vi "Create New IO Node.vi"(6 "Device Icon Name":string[](array[string]), 7 "Path to Analog Node Template":string="IONode\\Analog Input Node x.vi", 8 "error in":errorcluster, 9 "Device Alias":string, 10 "Values for Naming":T1={"Bus Number"=1, "Device Number"=1, "Channel Number"=1} {"Channel Number" min=1 step=1; "Device Number" min=1 step=1; "Bus Number" min=1 step=1}, 11 "Path to IO Node":path=path "D:/Documents/Projects/SPIAPI/IOEngineCode") -> (0 "error out":errorcluster, 2 "IO Node Name":string, 3 "Path to new IO Node":path)   [LabVIEW 2014, in "Initialization and IO Node Scripting.lvlib"]
uses:
  Initialization and IO Node Scripting.lvlib
  State Machine/Controls/Values for Naming.ctl
  Icon Editor/Icon Editor.llb/Icon Colors.ctl
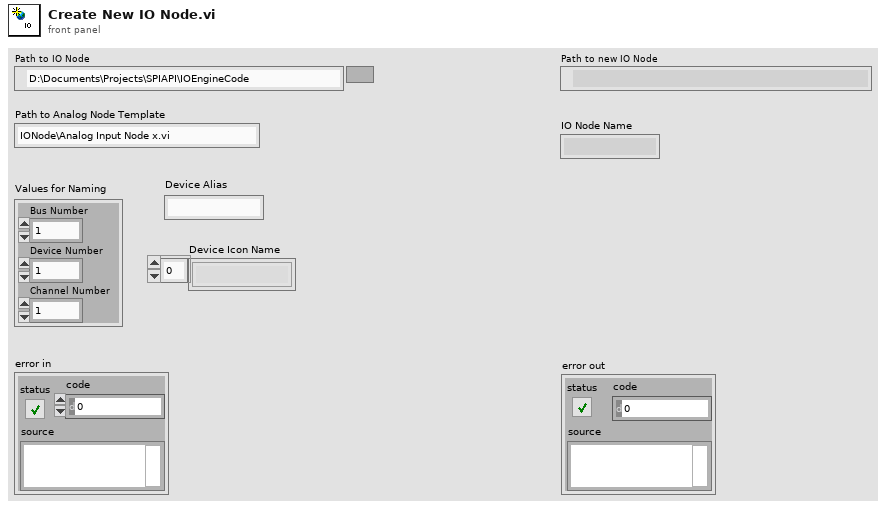
[diagram p1: front panel]
types:
  T1 = typedef "Initialization and IO Node Scripting.lvlib/Values for Naming.ctl" = cluster{"Bus Number":i32, "Device Number":i32, "Channel Number":i32}
  T2 = enum32{"invalid VI type", "Standard VI", "Control VI", "Global VI", "Polymorphic VI", "Configuration VI", "SubSystem", "Facade VI", "Method VI", "Statechart Diagram VI"}
  T3 = typedef "Initialization and IO Node Scripting.lvlib/Icon Colors.ctl" = cluster{"Text Color":u32, "Background Color":u32, "Border Color":u32}
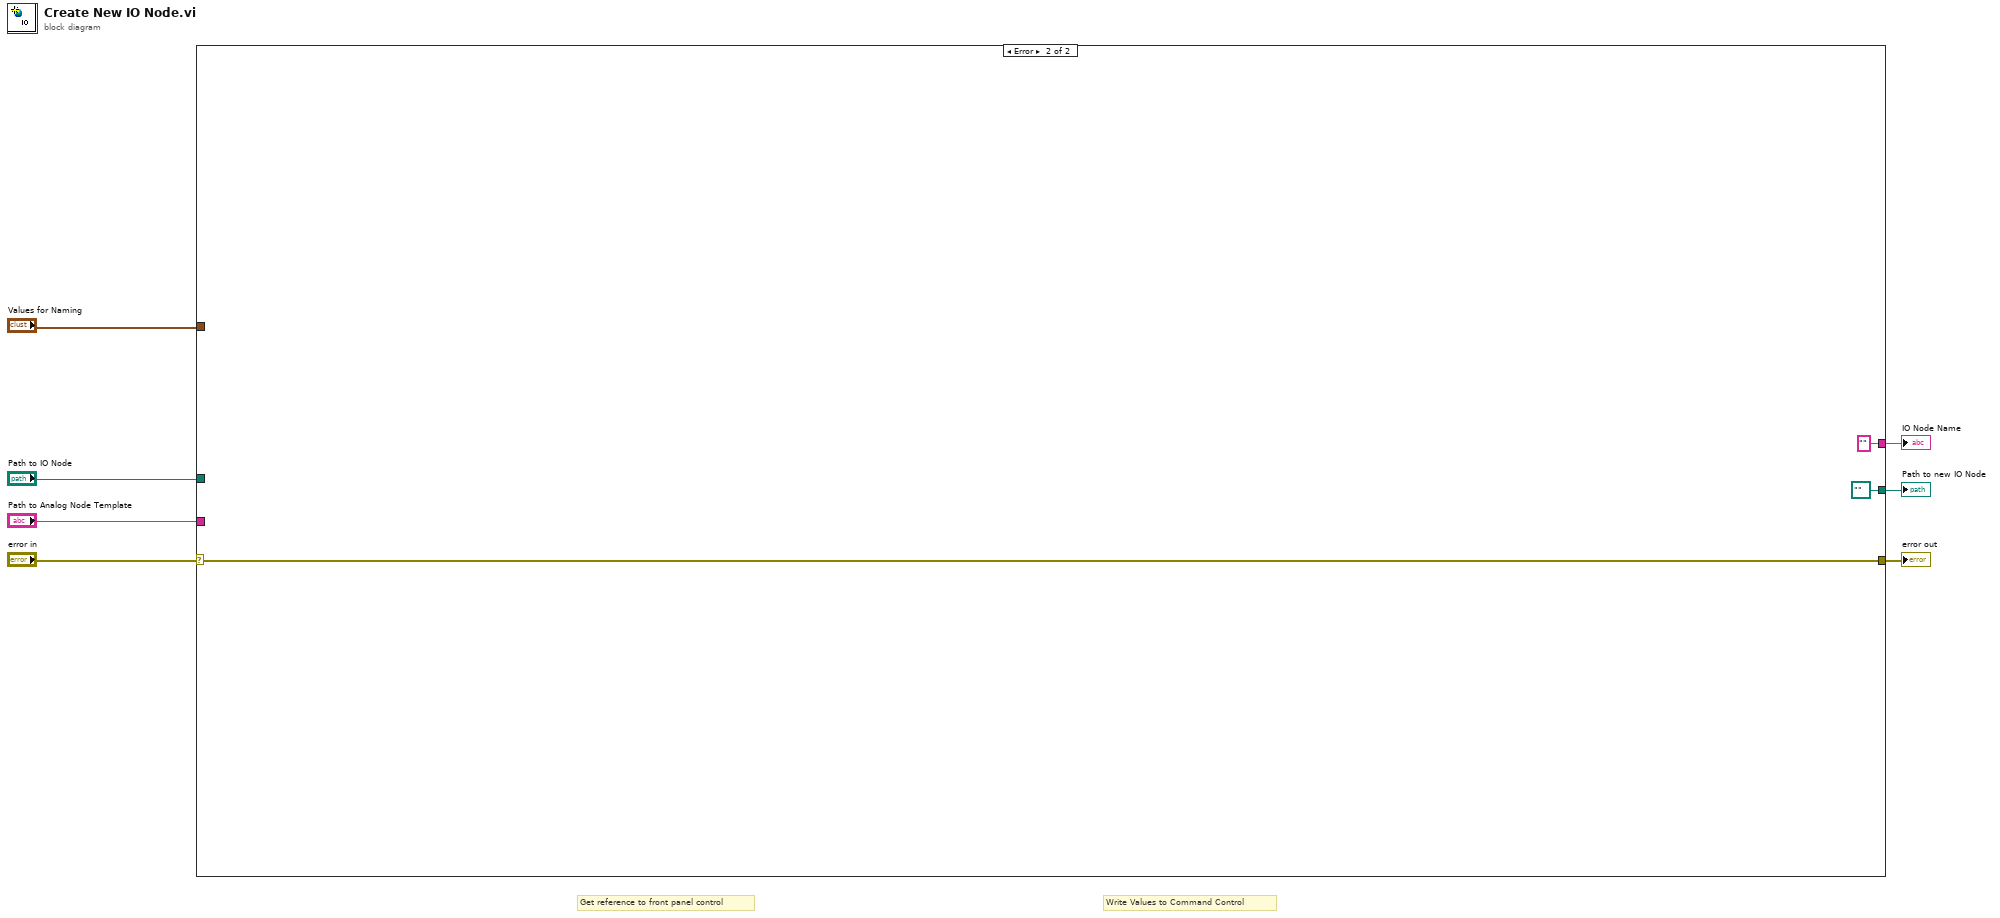
[diagram p0: block diagram]
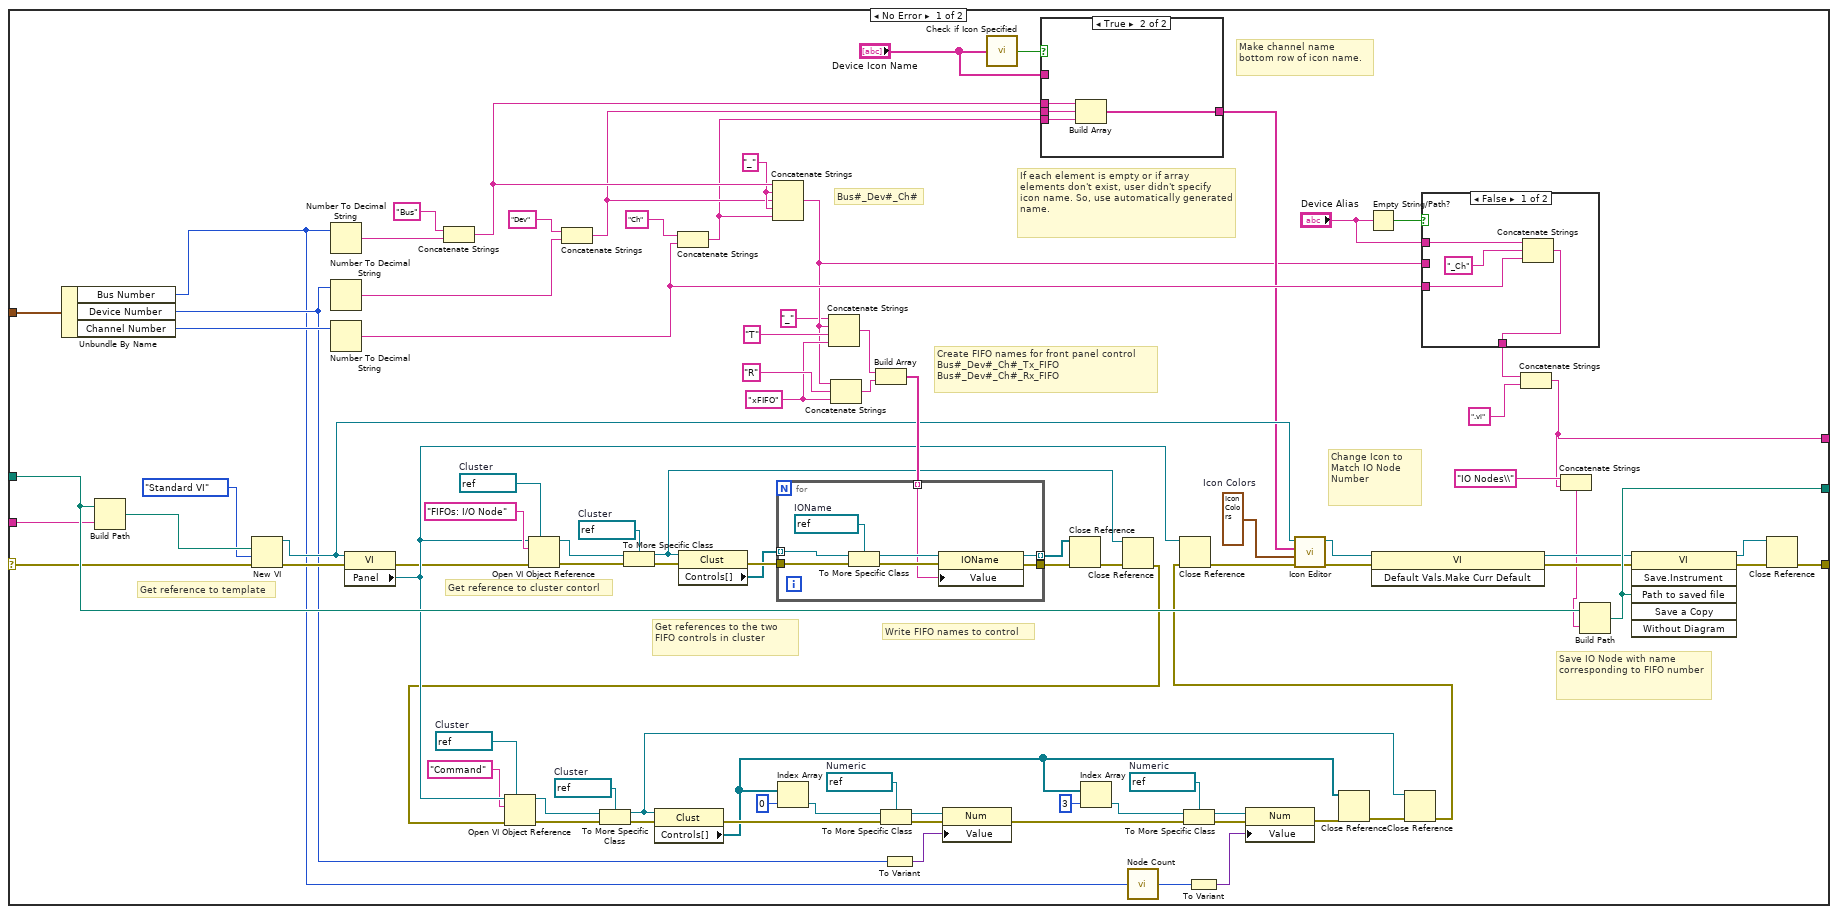
[diagram p2: hidden frame]
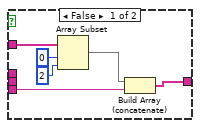
[diagram p4: hidden frame]
diagram:
  # "Get reference to front panel control"
  # "Write Values to Command Control"
  n1 = case shown="Error" "error in" {
    selector: "error in" -> [w79 w123]
    tunnel: "Path to IO Node" -> [w86 _]
    tunnel: [w84 path "" ("appended path")] -> w6
    tunnel: "Path to Analog Node Template" -> [w70 _]
    tunnel: "Values for Naming" -> [w69 _]
    tunnel: [w11 w123] -> w2
    tunnel: [w9 ""] -> w1
    frame No Error {
      w18 = "_" ("string")
      w41 = refnum<vi> refnum  # Numeric
      w52 = refnum<vi> refnum  # Numeric
      w55 = refnum<vi> refnum  # Cluster
      w54 = refnum<vi> refnum  # Cluster
      w71 = T3 {"Text Color"=0, "Background Color"=16448250, "Border Color"=16746744}  # Icon Colors
      w77 = "xFIFO" ("string")
      w95 = refnum<vi> refnum  # Cluster
      w97 = refnum<vi> refnum  # Cluster
      # "Make channel name bottom row of icon name."
      # "If each element is empty or if array elements don't exist, user didn't specify icon name. So, use automatically generated name."
      # "Get references to the two FIFO controls in cluster"
      # "Bus#_Dev#_Ch#"
      # "Change Icon to Match IO Node Number"
      # "Get reference to template"
      # "Create FIFO names for front panel control\nBus#_Dev#_Ch#_Tx_FIFO\nBus#_Dev#_Ch#_Rx_FIFO"
      # "Save IO Node with name corresponding to FIFO number"
      # "Write FIFO names to control"
      # "Get reference to cluster contorl"
      n2 = Unbundle By Name(w69) -> ("Bus Number"=w37:i32, "Device Number"=w39:i32, "Channel Number"=w68:i32)
      n3 = Build Path(base path=w86, name or relative path=w70) -> (appended path=w85:path)
      n4 = New VI(8:w79, 9:T2."Standard VI" ("vi type (standard vi)"), 10:w85) -> (0:w96:errorcluster, 3:w72:refnum<vi>)  [unwired: 4 in]
      n5 = Number To Decimal String(number=w37) -> (decimal integer string=w62:string)  [unwired: 1 in]
      n6 = Number To Decimal String(number=w39) -> (decimal integer string=w61:string)  [unwired: 1 in]
      n7 = Number To Decimal String(number=w68) -> (decimal integer string=w31:string)  [unwired: 1 in]
      n8 = property class="VI"(reference=w72, error in=w96) -> (error out=w63:errorcluster, "Panel"=w64:refnum<vi>)  [unwired: 1 out]
      n9 = Concatenate Strings("Bus" ("string"), w62) -> (w19:string)
      n10 = Open VI Object Reference(7:w97, 8:w63, 10:"FIFOs: I/O Node" ("name/order"), 11:w64) -> (0:w94:errorcluster, 3:w93:refnum<vi>)
      n11 = Concatenate Strings("Dev" ("string"), w61) -> (w17:string)
      n12 = To More Specific Class(target class=w95, reference=w93, error in=w94) -> (specific class reference=w25:refnum<vi>, error out=w26:errorcluster)
      n13 = Concatenate Strings("Ch" ("string"), w31) -> (w16:string)
      n14 = property class="Clust"(reference=w25, error in=w26) -> (error out=w88:errorcluster, "Controls[]"=w81:refnum<vi>[])  [unwired: 1 out]
      n15 = Concatenate Strings(w19, w18, w17, w18, w16) -> (w15:string)
      n16 = Concatenate Strings("_" ("string"), w15, "T" ("name or relative path"), w77) -> (w75:string)
      n17 = Concatenate Strings(w15, "R" ("name or relative path"), w77) -> (w74:string)
      n18 = Build Array(w75, w74) -> (w80:string[])
      n19 = for {
        tunnel: [w120] -> w90 mode=indexing
        tunnel: [w119] -> w89
        tunnel: w88 -> [w115]
        tunnel: w81 -> [w114] mode=indexing
        tunnel: w80 -> [w113] mode=indexing
        w116 = refnum<vi> refnum  # IOName
        n20 = To More Specific Class(target class=w116, reference=w114, error in=w115) -> (specific class reference=w117:refnum<vi>, error out=w118:errorcluster)
        n21 = property class="IOName"(reference=w117, error in=w118, "Value"=w113) -> (reference out=w120:refnum<vi>, error out=w119:errorcluster)
      }
      n22 = To Variant(anything=w39) -> (Variant=w47:variant)
      n23 = call "Check if Icon Specified.vi"("Device Icon Name"="Device Icon Name") -> ("No Icon Specified"=w24:bool)
      n24 = case shown="True" w24 {
        tunnel: w19 -> [_ w112]
        tunnel: w17 -> [_ w111]
        tunnel: w16 -> [w104 w110]
        tunnel: [w103 w109] -> w22
        tunnel: "Device Icon Name" -> [w108 _]
        frame False {
          n25 = Array Subset(array=w108, index=0, length=2) -> (w105:string[])
          n26 = Build Array (concatenate)(w105, w104) -> (w103:string[])
        }
        frame True {
          n27 = Build Array(w112, w111, w110) -> (w109:string[])
        }
      }
      n28 = Close Reference(reference=w90, error in (no error)=w89) -> (error out=w91:errorcluster)
      n29 = Close Reference(reference=w25, error in (no error)=w91) -> (error out=w33:errorcluster)
      n30 = Open VI Object Reference(7:w54, 8:w33, 10:"Command" ("name/order"), 11:w64) -> (0:w57:errorcluster, 3:w58:refnum<vi>)
      n31 = To More Specific Class(target class=w55, reference=w58, error in=w57) -> (specific class reference=w53:refnum<vi>, error out=w56:errorcluster)
      n32 = property class="Clust"(reference=w53, error in=w56) -> (error out=w60:errorcluster, "Controls[]"=w35:refnum<vi>[])  [unwired: 1 out]
      n33 = Index Array(array=w35, index=0) -> (element=w50:refnum<vi>)
      n34 = To More Specific Class(target class=w52, reference=w50, error in=w60) -> (specific class reference=w49:refnum<vi>, error out=w48:errorcluster)
      n35 = property class="Num"(reference=w49, error in=w48, "Value"=w47) -> (error out=w40:errorcluster)  [unwired: 1 out]
      n36 = Index Array(array=w35, index=3) -> (element=w43:refnum<vi>)
      n37 = call "Node Count.vi"("Bus Number in"=w37) -> ("Node Number"=w38:i32)
      n38 = To More Specific Class(target class=w41, reference=w43, error in=w40) -> (specific class reference=w44:refnum<vi>, error out=w45:errorcluster)
      n39 = To Variant(anything=w38) -> (Variant=w46:variant)
      n40 = property class="Num"(reference=w44, error in=w45, "Value"=w46) -> (error out=w34:errorcluster)  [unwired: 1 out]
      n41 = Close Reference(reference=w35, error in (no error)=w34) -> (error out=w36:errorcluster)
      n42 = Empty String/Path?(string/path="Device Alias") -> (empty?=w21:bool)
      n43 = Close Reference(reference=w53, error in (no error)=w36) -> (error out=w32:errorcluster)
      n44 = Close Reference(reference=w64, error in (no error)=w32) -> (error out=w73:errorcluster)
      n45 = call "Icon Editor.vi"("Error In"=w73, "Icon Colors"=w71, "Text Array"=w22, "Reference to VI"=w72) -> ("Error Out"=w30:errorcluster, "Reference to VI"=w29:refnum<vi>)  [unwired: 6 in]
      n46 = invoke class="VI" method="Default Vals.Make Curr Default"(reference=w29, error in=w30) -> (reference out=w27:refnum<vi>, error out=w28:errorcluster)  [unwired: 1 in, 1 out]
      n47 = case shown="False" w21 {
        tunnel: [w98 w102] -> w13
        tunnel: w31 -> [w100 _]
        tunnel: "Device Alias" -> [w99 _]
        tunnel: w15 -> [_ w102]
        frame False {
          n48 = Concatenate Strings(w99, "_Ch" ("string"), w100) -> (w98:string)
        }
        frame True {
        }
      }
      n49 = Concatenate Strings(w13, ".vi" ("string")) -> (w9:string)
      n50 = Concatenate Strings("IO Nodes\\" ("string"), w9) -> (w8:string)
      n51 = Build Path(base path=w86, name or relative path=w8) -> (appended path=w84:path)
      n52 = invoke class="VI" method="Save.Instrument"(reference=w27, error in=w28, "Path to saved file"=w84) -> (reference out=w83:refnum<vi>, error out=w87:errorcluster)  [unwired: 3 in, 4 out]
      n53 = Close Reference(reference=w83, error in (no error)=w87) -> (error out=w11:errorcluster)
    }
    frame Error {
    }
  }
  "error out" <- w2
  "Path to new IO Node" <- w6
  "IO Node Name" <- w1
